vi "Decode bool.vi"(10 "Wire Type":T1, 11 "Data":u8[](array[numeric]) format="%.0x") -> (2 "error out":errorcluster, 3 "bool":bool)   [LabVIEW 2020, in "LV-Proto.lvlib"]
uses:
  LV-Proto.lvlib
  Wire Type.ctl
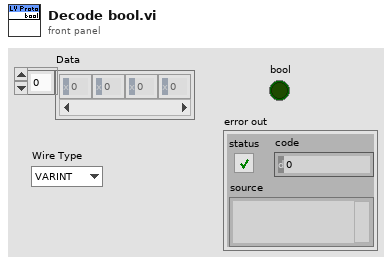
[diagram p1: front panel]
types:
  T1 = typedef "LV-Proto.lvlib/Wire Type.ctl" = enum8{"VARINT", "I64", "LEN", "SGROUP (Deprecated)", "EGROUP (Deprecated)", "I32"}
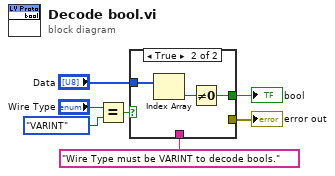
[diagram p0: block diagram]
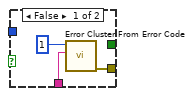
[diagram p2: hidden frame]
diagram:
  n1 = Equal?(x="Wire Type", y=Wire_Type."VARINT") -> (x = y?=w3:bool)
  n2 = case shown="True" w3 {
    tunnel: [_ w13] -> w7
    tunnel: "Data" -> [_ w12]
    tunnel: [w9 _] -> w2
    tunnel: "Wire Type must be VARINT to decode bools." -> [w8 _]
    frame False {
      n3 = call <vilib>:"Error Cluster From Error Code.vi"("error message (\"\")"=w8, "error code (0)"=1) -> ("error out"=w9:errorcluster)  [unwired: 7 in]
    }
    frame True {
      n4 = Index Array(array=w12) -> (element=w11:u8)  [unwired: 1 in]
      n5 = Not Equal To 0?(x=w11) -> (x != 0?=w13:bool)
    }
  }
  "bool" <- w7
  "error out" <- w2
